vi "Paste From Clipboard.vi"   [LabVIEW 2023]
doc: "Demonstrates the Paste method in VI Scripting, which pastes the current contents of the clipboard into a VI. It has the same effect as choosing Edit > Paste from the user interface."
uses:
  <vilib>/Utility/miscctls.llb/LVPositionTypeDef.ctl
panel:
  # "Overview: Demonstrates the Paste method in VI Scripting, which pastes the current contents of the clipboard into a VI.\nInstructions:\n1. Open a new VI.\n2. Drop several items on the block diagram of the new VI.\n3. Highlight all of the items you dropped and choose Edit > Copy from the menu bar. This places those items on the system clipboard.\n4. Open the block diagram of Test - Selection List Target.vi.\n5. Run this VI. The contents of the system clipboard will be pasted into the diagram of Test - Selection List Target.vi."
types:
  T1 = typedef "LVPositionTypeDef.ctl" = cluster{"Left":i32, "Top":i32}
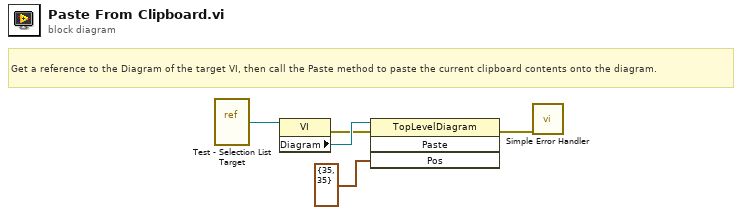
[diagram p0: block diagram]
diagram:
  # "Get a reference to the Diagram of the target VI, then call the Paste method to paste the current clipboard contents onto the diagram."
  n1 = vi-ref "Test - Selection List Target.vi"() -> (w5:refnum<vi>)
  n2 = property class="VI"(reference=w5) -> (error out=w3:errorcluster, "Diagram"=w4:refnum<vi>)  [unwired: 1 in, 1 out]
  n3 = invoke class="TopLevelDiagram" method="Paste"(reference=w4, error in=w3, "Pos"=T1 {"Left"=35, "Top"=35} ("Position")) -> (error out=w2:errorcluster)  [unwired: 1 in, 3 out]
  n4 = call <vilib>:"Simple Error Handler.vi"("error in (no error)"=w2) -> ()  [unwired: 4 in, 5 out]
